vi "Get Devices.vi"(8 "error in (no error)":errorcluster) -> (0 "error out":errorcluster, 2 "Device Names":string[](array[string]))   [LabVIEW 2020, in "MIDIllan.lvlib" / "midi out.lvclass"]
doc: "Gets the names of all MIDI output devices."
uses:
  midi out.lvclass
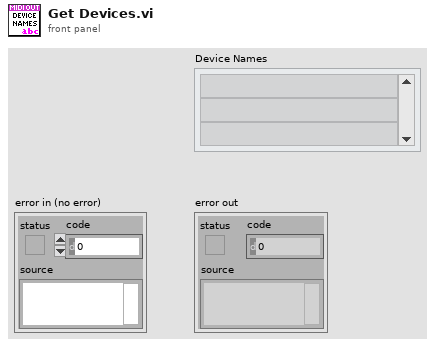
[diagram p1: front panel]
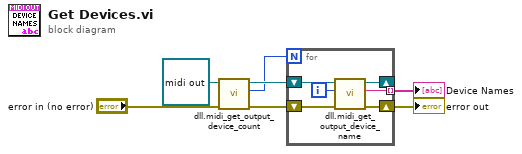
[diagram p0: block diagram]
diagram:
  n1 = call "dll.midi_get_output_device_count.vi"("error in (no error)"="error in (no error)", "midi out in"=refnum<class "midi out.lvclass"> refnum) -> ("error out"=w4:errorcluster, "Device Count"=w5:i32, "midi out"=w6:refnum<class "midi out.lvclass">)  [unwired: 7 in]
  n2 = for {
    N: w5 -> [_]
    shift-right: [w10] -> _
    shift-left: w6 -> [w12]
    shift-right: [w9] -> w3
    shift-left: w4 -> [w11]
    tunnel: [w8] -> w1 mode=indexing
    i -> [w13]
    n3 = call "dll.midi_get_output_device_name.vi"("error in (no error)"=w11, "Device Index"=w13, "midi out in"=w12) -> ("error out"=w9:errorcluster, "Name"=w8:string, "midi out"=w10:refnum<class "midi out.lvclass">)  [unwired: 6 in]
  }
  "error out" <- w3
  "Device Names" <- w1
